vi "Load Settings from XML.vi"(8 "error in (no error)":errorcluster, 11 "Settings in":T1={"Hardware Configuration"={"COM Port"="", "Reference Distance"=0.0, "Sensor SN"=""}, "Logging Configuration"={"Log File Base Path"=path "", "Datafile Ref"=refnum, "Database Ref"=refnum}, "UI Refs"={"Start Ref"=refnum, "Settings Ref"=refnum, "Stop Ref"=refnum, "Exit Ref"=refnum, "Status Ref"=refnum, "Data Ref"=refnum, "StatusBox Ref"=refnum, "Location Ref"=refnum, "Operator Ref"=refnum, "Time Ref"=refnum, "Test in Progess Ref"=refnum}, "Calibration Data"={"calibrationID"=0, "operatorID"=0, "sensorID"=0, "start_time"="", "end_time"="", "offset"=0.0, "offset_units"="", "ring_time"=0.0, "error"=0.0, "Passed"=0, "data_storage_location"="", "comments"=""}, "Time Elapsed"=0, "Samples Required"=480} {"Hardware Configuration"."Reference Distance" format="%.3g"}) -> (0 "error out":errorcluster, 3 "Settings out":T1={"Hardware Configuration"={"COM Port"="", "Reference Distance"=0.0, "Sensor SN"=""}, "Logging Configuration"={"Log File Base Path"=path "", "Datafile Ref"=refnum, "Database Ref"=refnum}, "UI Refs"={"Start Ref"=refnum, "Settings Ref"=refnum, "Stop Ref"=refnum, "Exit Ref"=refnum, "Status Ref"=refnum, "Data Ref"=refnum, "StatusBox Ref"=refnum, "Location Ref"=refnum, "Operator Ref"=refnum, "Time Ref"=refnum, "Test in Progess Ref"=refnum}, "Calibration Data"={"calibrationID"=0, "operatorID"=0, "sensorID"=0, "start_time"="", "end_time"="", "offset"=0.0, "offset_units"="", "ring_time"=0.0, "error"=0.0, "Passed"=0, "data_storage_location"="", "comments"=""}, "Time Elapsed"=0, "Samples Required"=480} {"Hardware Configuration"."Reference Distance" format="%.3g"})   [LabVIEW 2018, in "Settings.lvlib"]
doc: "Attempts to load previous user specified settings from an XML file.\n\nThis VI will not generate an error. If a suitable XML file can't be loaded and parsed then it will simply return the default settings."
uses:
  Settings.lvlib
  Settings.ctl
  Acquisition/Hardware Configuration.ctl
  Logging/Logging Configuration.ctl
  <vilib>/addons/database/Connection.llb/Conn ObjectReference.ctl
  Controls/Location Ring.ctl
  Controls/Time Remaining.ctl
  <vilib>/Utility/xml.llb/Read From XML File(string).vi
  <vilib>/Utility/xml.llb/Write to XML File(string).vi
  Acquisition/Acquisition.lvlib
  Logging/Logging.lvlib
  <vilib>/addons/database/NI_Database_API.lvlib
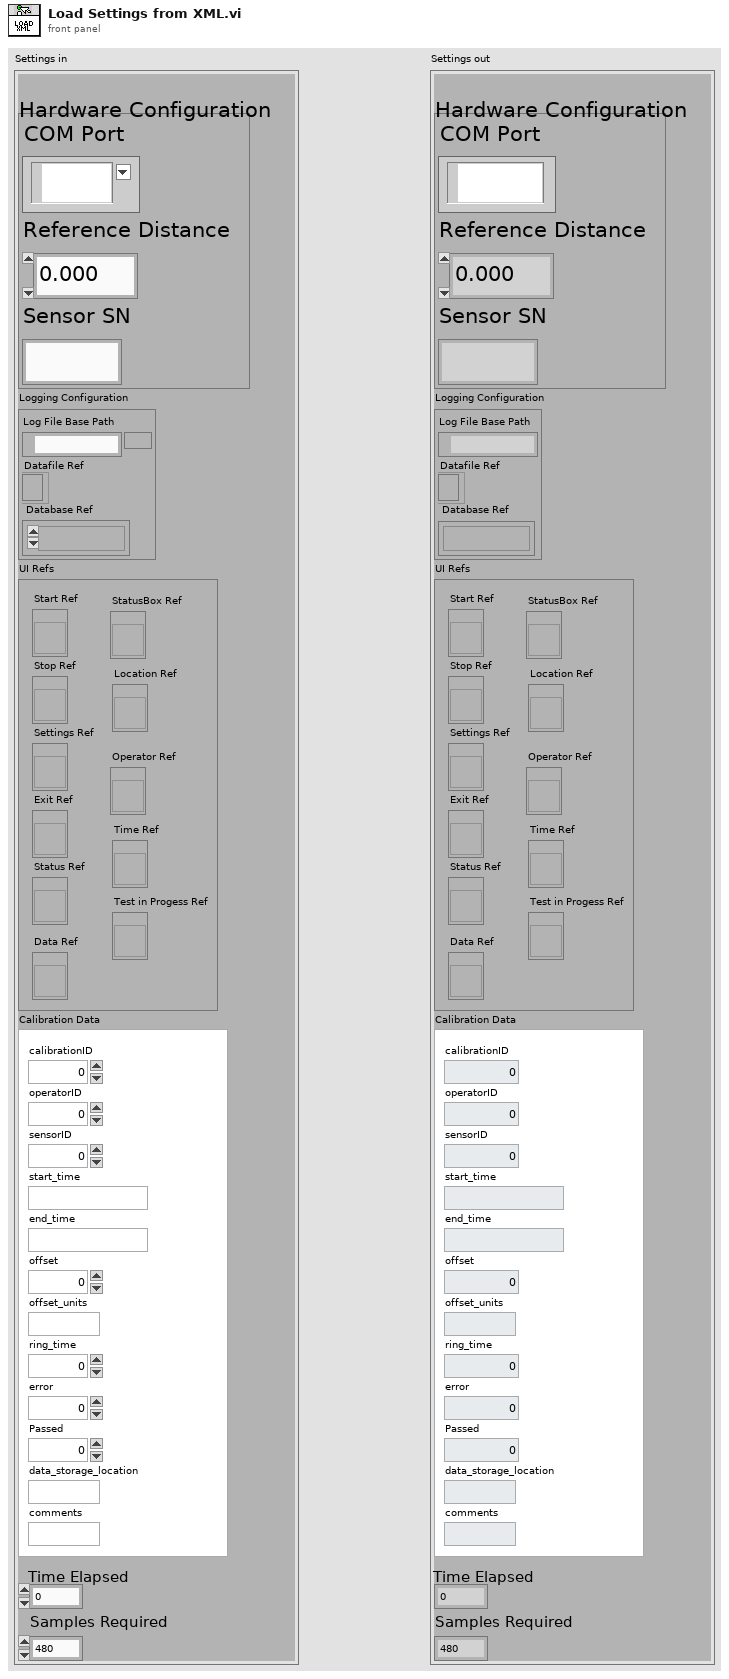
[diagram p1: front panel]
types:
  T1 = typedef "Settings.lvlib/Settings.ctl" = cluster{"Hardware Configuration":T2, "Logging Configuration":T3, "UI Refs":cluster{"Start Ref":refnum<vi>, "Settings Ref":refnum<vi>, "Stop Ref":refnum<vi>, "Exit Ref":refnum<vi>, "Status Ref":refnum<vi>, "Data Ref":refnum<vi>, "StatusBox Ref":refnum<vi>, "Location Ref":refnum<vi>, "Operator Ref":refnum<vi>, "Time Ref":refnum<vi>, "Test in Progess Ref":refnum<vi>}, "Calibration Data":cluster{"calibrationID":u16, "operatorID":u16, "sensorID":u16, "start_time":string, "end_time":string, "offset":dbl, "offset_units":string, "ring_time":dbl, "error":dbl, "Passed":u8, "data_storage_location":string, "comments":string}, "Time Elapsed":u16, "Samples Required":u16}
  T2 = typedef "Acquisition.lvlib/Hardware Configuration.ctl" = cluster{"COM Port":refnum<visa-resource-name>, "Reference Distance":dbl, "Sensor SN":string}
  T3 = typedef "Logging.lvlib/Logging Configuration.ctl" = cluster{"Log File Base Path":path, "Datafile Ref":refnum<file>, "Database Ref":T4}
  T4 = typedef "NI_Database_API.lvlib/Conn ObjectReference.ctl" = refnum<k1>
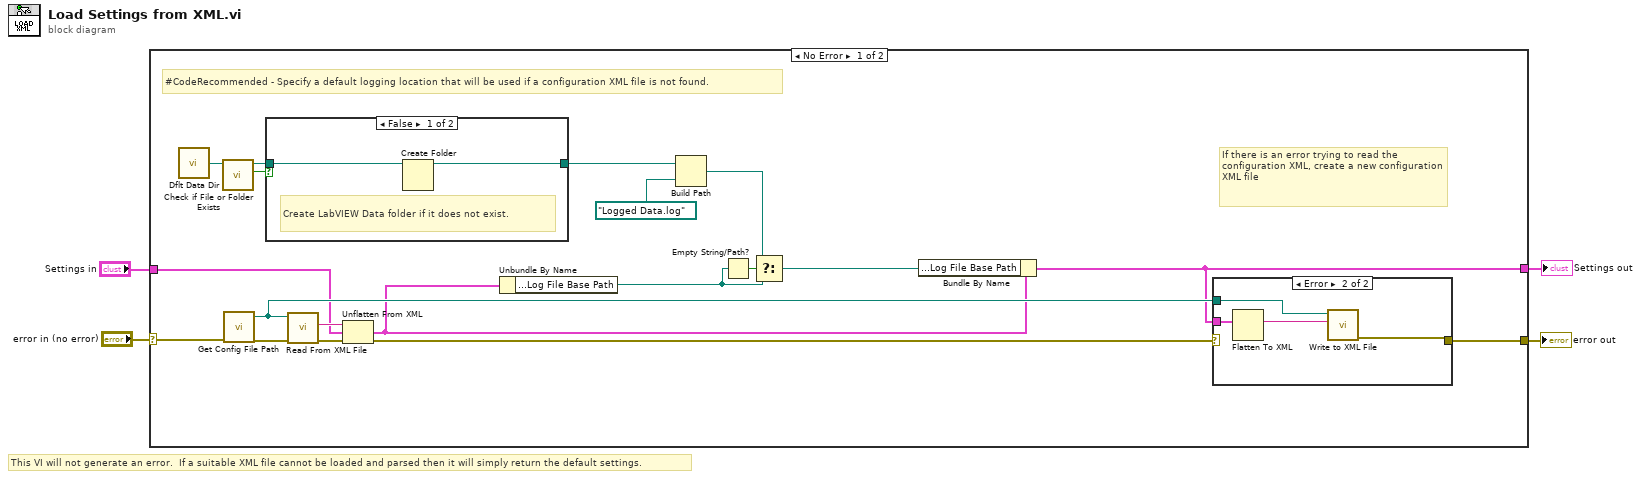
[diagram p0: block diagram]
diagram:
  # "This VI will not generate an error.  If a suitable XML file cannot be loaded and parsed then it will simply return the default settings."
  n1 = case shown="No Error" "error in (no error)" {
    selector: "error in (no error)" -> [w21 w32]
    tunnel: "Settings in" -> [w16 w33]
    tunnel: [w10 w33] -> w2
    tunnel: [w5 w32] -> w1
    frame No Error {
      # "If there is an error trying to read the configuration XML, create a new configuration XML file"
      # "#CodeRecommended - Specify a default logging location that will be used if a configuration XML file is not found."
      n2 = call <vilib>:"Dflt Data Dir.vi"() -> ("App:Default Data Directory"=w9:path)
      n3 = call <vilib>:"Check if File or Folder Exists.vi"("path"=w9) -> ("file or folder exists?"=w8:bool, "dup path"=w7:path)  [unwired: 8 in, 1 out]
      n4 = call "Get Config File Path.vi"("error in (no error)"=w21) -> ("error out"=w23:errorcluster, "XML File Path"=w19:path)  [unwired: 9 in]
      n5 = case shown="False" w8 {
        tunnel: w7 -> [w25 w26]
        tunnel: [w24 w26] -> w6
        frame False {
          # "Create LabVIEW Data folder if it does not exist."
          n6 = Create Folder(path (use dialog)=w25) -> (created path=w24:path)  [unwired: 2 in, 2 out]
        }
        frame True {
        }
      }
      n7 = call-poly <vilib>:"Read From XML File.vi"("error in (no error)"=w23, "XML File Path"=w19) -> ("error out"=w18:errorcluster, "XML Elements"=w22:string)  [unwired: 7 in, 1 out]
      n8 = Unflatten From XML(xml string=w22, type=w16, error in (no error)=w18) -> (value=w12:T1, error out=w17:errorcluster)
      n9 = Unbundle By Name(w12) -> ("Logging Configuration.Log File Base Path"=w14:path)
      n10 = Build Path(base path=w6, name or relative path=path "Logged Data.log" ("App:Default Data Directory")) -> (appended path=w13:path)
      n11 = Empty String/Path?(string/path=w14) -> (empty?=w15:bool)
      n12 = Select(t=w13, s=w15, f=w14) -> (s? t:f=w11:path)
      n13 = Bundle By Name(cluster=w12, "Logging Configuration.Log File Base Path"=w11) -> (w10:T1)
      n14 = case shown="Error" w17 {
        selector: w17 -> [w27 _]
        tunnel: w10 -> [_ w31]
        tunnel: w19 -> [_ w29]
        tunnel: [w27 w28] -> w5
        frame No Error {
        }
        frame Error {
          n15 = Flatten To XML(anything=w31) -> (xml string=w30:string)
          n16 = call-poly <vilib>:"Write to XML File.vi"("XML Input"=w30, "XML File Path"=w29) -> ("error out"=w28:errorcluster)  [unwired: 7 in, 2 out]
        }
      }
    }
    frame Error {
    }
  }
  "error out" <- w1
  "Settings out" <- w2
